vi "traverse controls.vi"(6 "controls":refnum<vi>[](array[refnum]), 8 "error in (no error)":errorcluster, 11 "controls map in":map{string, T1}(c390)) -> (0 "error out":errorcluster, 3 "controls map out":map{string, T1}(c390))   [LabVIEW 2024, in "controls manager.lvlib"]
uses:
  controls manager.lvlib
  control.ctl
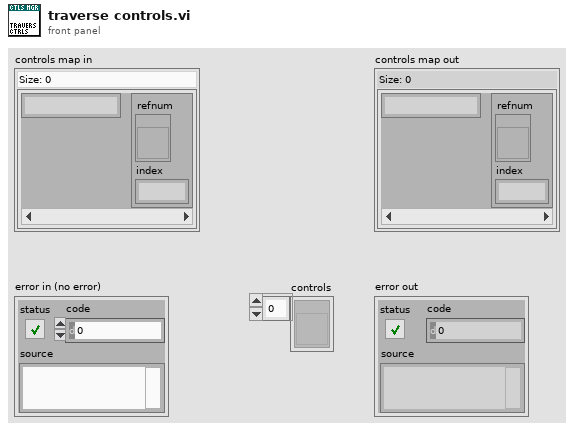
[diagram p1: front panel]
types:
  T1 = typedef "controls manager.lvlib/control.ctl" = cluster{"refnum":refnum<vi>, "index":i32}
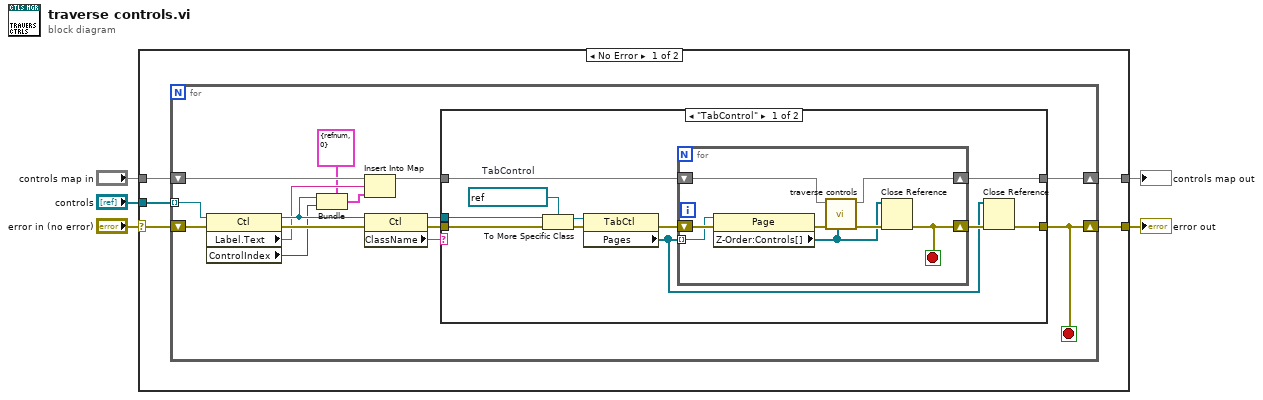
[diagram p0: block diagram]
diagram:
  n1 = case shown="No Error" "error in (no error)" {
    selector: "error in (no error)" -> [w8 w48]
    tunnel: [w10 w48] -> w5
    tunnel: "controls" -> [w9 _]
    tunnel: "controls map in" -> [w7 w47]
    tunnel: [w6 w47] -> w1
    frame No Error {
      n2 = for {
        tunnel: w9 -> [w17] mode=indexing
        shift-right: [w13] -> w6
        shift-left: w7 -> [w25]
        shift-right: [w20] -> w10
        shift-left: w8 -> [w18]
        stop <- w20 stop-if-true
        n3 = property on="Property Node" class="Ctl"(reference=w17, error in=w18) -> (reference out=w16:refnum<vi>, error out=w24:errorcluster, "Label.Text"=w12:string, "ControlIndex"=w15:i32)
        n4 = Bundle(cluster=T1 {"refnum"=refnum, "index"=0}, "refnum"=w16, "index"=w15) -> (w14:T1)
        n5 = Insert Into Map(map in=w25, key=w12, value=w14) -> (map out=w19:map{string, T1})  [unwired: 2 out]
        n6 = property class="Ctl"(reference=w16, error in=w24) -> (reference out=w22:refnum<vi>, error out=w21:errorcluster, "ClassName"=w23:string)
        n7 = case shown="\"TabControl\"" w23 {
          tunnel: w22 -> [w27 _]
          tunnel: [w35 w46] -> w13
          tunnel: w19 -> [w28 w46]
          tunnel: [w30 w45] -> w20
          tunnel: w21 -> [w26 w45]
          frame "TabControl" {
            w31 = refnum<vi> refnum  # TabControl
            n8 = To More Specific Class(target class=w31, reference=w27, error in=w26) -> (specific class reference=w33:refnum<vi>, error out=w32:errorcluster)
            n9 = property on="Property Node" class="TabCtl"(reference=w33, error in=w32) -> (error out=w36:errorcluster, "Pages"=w29:refnum<vi>[])  [unwired: 1 out]
            n10 = for {
              tunnel: w29 -> [w41] mode=indexing
              shift-right: [w37] -> w35
              shift-left: w28 -> [w38]
              shift-right: [w40] -> w34
              shift-left: w36 -> [w44]
              stop <- w40 stop-if-true
              n11 = property on="Property Node" class="Page"(reference=w41, error in=w44) -> (error out=w43:errorcluster, "Z-Order:Controls[]"=w39:refnum<vi>[])  [unwired: 1 out]
              n12 = call "traverse controls.vi"("controls"=w39, "error in (no error)"=w43, "controls map in"=w38) -> ("error out"=w42:errorcluster, "controls map out"=w37:map{string, T1})  [unwired: 7 in]
              n13 = Close Reference(reference=w39, error in (no error)=w42) -> (error out=w40:errorcluster)
            }
            n14 = Close Reference(reference=w29, error in (no error)=w34) -> (error out=w30:errorcluster)
          }
          frame Default {
          }
        }
      }
    }
    frame Error {
    }
  }
  "error out" <- w5
  "controls map out" <- w1
